vi "Read Laser Power.vi"(8 "error in (no error)":errorcluster, 10 "Power":dbl, 11 "Application in":refnum<class "Application.lvclass">) -> (0 "error out":errorcluster, 3 "Application out":refnum<class "Application.lvclass">)   [LabVIEW 2023, in "Application.lvlib" / "Application.lvclass"]
uses:
  Application.lvclass
  Application.lvclass/Application.ctl
  User Interface/Main Window Messages/Read Laser Power Msg/Read Laser Power Msg.lvclass/Read Laser Power Msg.ctl
  <vilib>/ActorFramework/Message Enqueuer/Message Enqueuer.lvclass/Message Enqueuer.ctl
  <vilib>/ActorFramework/Message Enqueuer/Enqueue.vi
  User Interface/Main Window Messages/Read Laser Power Msg/Read Laser Power Msg.lvclass
  C:/Program Files/National Instruments/LabVIEW 2023/vi.lib/ActorFramework/Message/Message.lvclass
  Resources/GLOBAL/GLOBAL Experiment Metadata.vi
  <vilib>/ActorFramework/Message Priority Queue/Priority Enqueue.vi
  Mode.ctl
  Application.lvlib
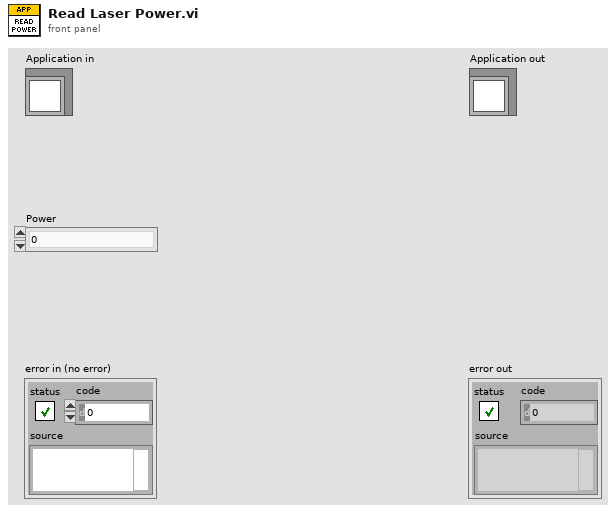
[diagram p1: front panel]
types:
  T1 = typedef "Application.lvlib/Mode.ctl" = enum16{"Idle", "Cancel", "Live", "Stream", "Autofocus", "Z-Stack", "Montage", "Saving", "Stage Scan", "Laser Adjust"}
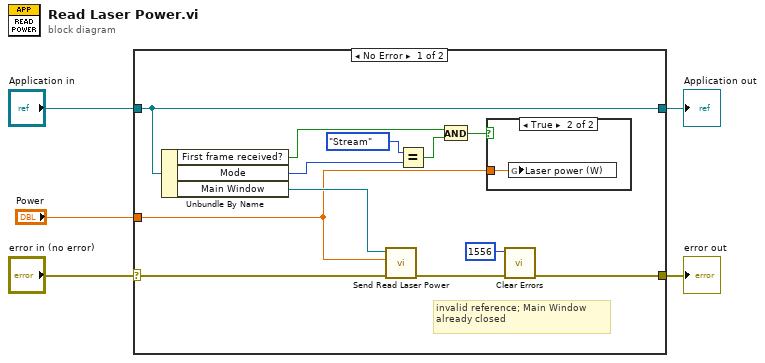
[diagram p0: block diagram]
diagram:
  n1 = case shown="No Error" "error in (no error)" {
    selector: "error in (no error)" -> [w16 w20]
    tunnel: [w12 w20] -> w4
    tunnel: [w17 w19] -> w2
    tunnel: "Application in" -> [w17 w19]
    tunnel: "Power" -> [w14 _]
    frame No Error {
      # "invalid reference; Main Window already closed"
      n2 = Unbundle By Name(w17) -> ("First frame received?"=w9:bool, "Mode"=w7:T1, "Main Window"=w15:refnum<class "Message Enqueuer.lvclass">)
      n3 = call "Send Read Laser Power.vi"("error in (no error)"=w16, "Power"=w14, "Message Enqueuer"=w15) -> ("error out"=w13:errorcluster)  [unwired: 7 in, 1 out]
      n4 = Equal?(x=Mode."Stream" ("y"), y=w7) -> (x = y?=w8:bool)
      n5 = And(x=w9, y=w8) -> (x .and. y?=w10:bool)
      n6 = case shown="True" w10 {
        tunnel: w14 -> [_ w18]
        frame False {
        }
        frame True {
          n7 = global write "GLOBAL Experiment Metadata.vi" "Laser power (W)"(w18) -> ()
        }
      }
      n8 = call <vilib>:"Clear Errors.vi"("error in (no error)"=w13, "specific error code to clear (0: all)"=1556) -> ("error out"=w12:errorcluster)  [unwired: 4 in, 1 out]
    }
    frame Error {
    }
  }
  "error out" <- w4
  "Application out" <- w2
